vi "CODMn报警信息.vi"(11 "报警簇":T1) -> (3 "CODMN报警信息":string)   [LabVIEW 2016, in "斯坦道CODMn.lvlib"]
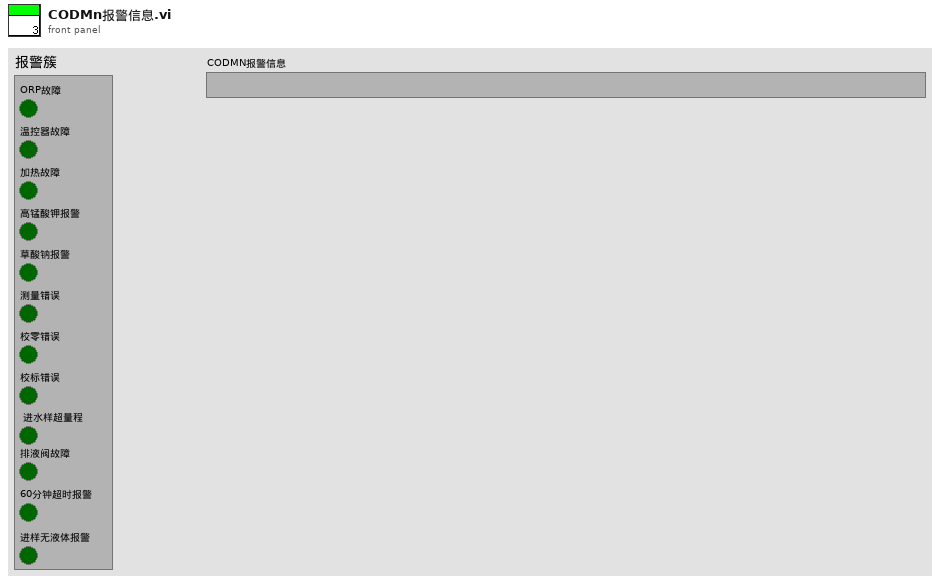
[diagram p1: front panel]
types:
  T1 = cluster{"ORP故障":bool, "温控器故障":bool, "加热故障":bool, "高锰酸钾报警":bool, "草酸钠报警":bool, "测量错误":bool, "校零错误":bool, "校标错误":bool, " 进水样超量程":bool, "排液阀故障":bool, "60分钟超时报警":bool, "进样无液体报警":bool}
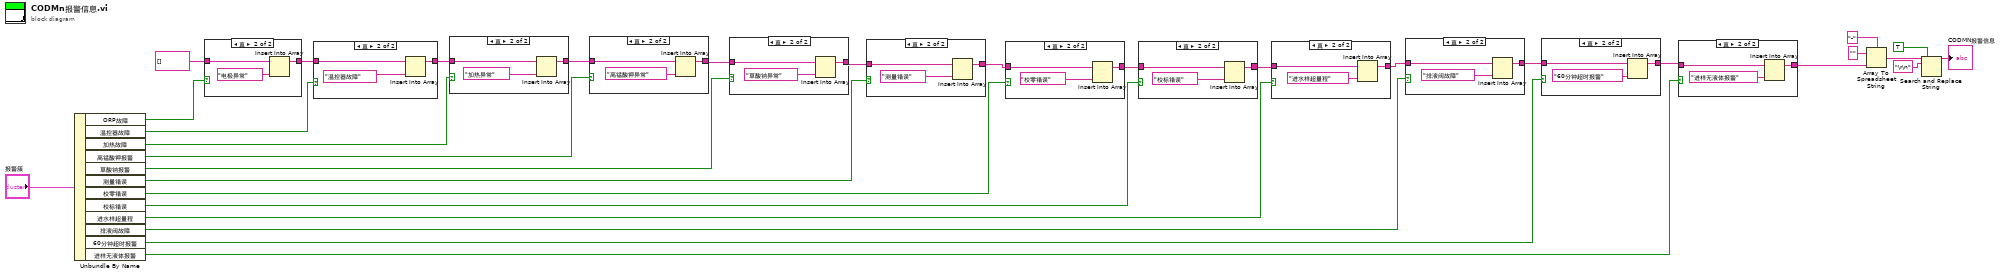
[diagram p0: block diagram]
diagram:
  n1 = Unbundle By Name("报警簇") -> ("ORP故障"=w32:bool, "温控器故障"=w31:bool, "加热故障"=w28:bool, "高锰酸钾报警"=w12:bool, "草酸钠报警"=w11:bool, "测量错误"=w10:bool, "校零错误"=w9:bool, "校标错误"=w8:bool, "进水样超量程"=w7:bool, "排液阀故障"=w6:bool, "60分钟超时报警"=w4:bool, "进样无液体报警"=w2:bool)
  n2 = case shown="真" w32 {
    tunnel: string[] [] -> [w33 w35]
    tunnel: [w33 w34] -> w29
    frame False {
    }
    frame True {
      n3 = Insert Into Array(array=w35, new element="电极异常" ("组合框")) -> (w34:string[])  [unwired: 1 in]
    }
  }
  n4 = case shown="真" w31 {
    tunnel: w29 -> [w37 w40]
    tunnel: [w37 w39] -> w25
    frame False {
    }
    frame True {
      n5 = Insert Into Array(array=w40, new element="温控器故障" ("组合框")) -> (w39:string[])  [unwired: 1 in]
    }
  }
  n6 = case shown="真" w28 {
    tunnel: w25 -> [w41 w43]
    tunnel: [w41 w44] -> w13
    frame False {
    }
    frame True {
      n7 = Insert Into Array(array=w43, new element="加热异常" ("组合框")) -> (w44:string[])  [unwired: 1 in]
    }
  }
  n8 = case shown="真" w12 {
    tunnel: w13 -> [w45 w47]
    tunnel: [w45 w48] -> w14
    frame False {
    }
    frame True {
      n9 = Insert Into Array(array=w47, new element="高锰酸钾异常" ("组合框")) -> (w48:string[])  [unwired: 1 in]
    }
  }
  n10 = case shown="真" w11 {
    tunnel: w14 -> [w49 w51]
    tunnel: [w49 w52] -> w15
    frame False {
    }
    frame True {
      n11 = Insert Into Array(array=w51, new element="草酸钠异常" ("组合框")) -> (w52:string[])  [unwired: 1 in]
    }
  }
  n12 = case shown="真" w10 {
    tunnel: w15 -> [w53 w55]
    tunnel: [w53 w56] -> w16
    frame False {
    }
    frame True {
      n13 = Insert Into Array(array=w55, new element="测量错误" ("组合框")) -> (w56:string[])  [unwired: 1 in]
    }
  }
  n14 = case shown="真" w9 {
    tunnel: w16 -> [w57 w59]
    tunnel: [w57 w60] -> w19
    frame False {
    }
    frame True {
      n15 = Insert Into Array(array=w59, new element="校零错误" ("组合框")) -> (w60:string[])  [unwired: 1 in]
    }
  }
  n16 = case shown="真" w8 {
    tunnel: w19 -> [w61 w63]
    tunnel: [w61 w64] -> w18
    frame False {
    }
    frame True {
      n17 = Insert Into Array(array=w63, new element="校标错误" ("组合框")) -> (w64:string[])  [unwired: 1 in]
    }
  }
  n18 = case shown="真" w7 {
    tunnel: w18 -> [w65 w67]
    tunnel: [w65 w68] -> w17
    frame False {
    }
    frame True {
      n19 = Insert Into Array(array=w67, new element="进水样超量程" ("组合框")) -> (w68:string[])  [unwired: 1 in]
    }
  }
  n20 = case shown="真" w6 {
    tunnel: w17 -> [w69 w71]
    tunnel: [w69 w72] -> w5
    frame False {
    }
    frame True {
      n21 = Insert Into Array(array=w71, new element="排液阀故障" ("组合框")) -> (w72:string[])  [unwired: 1 in]
    }
  }
  n22 = case shown="真" w4 {
    tunnel: w5 -> [w73 w74]
    tunnel: [w73 w76] -> w3
    frame False {
    }
    frame True {
      n23 = Insert Into Array(array=w74, new element="60分钟超时报警" ("组合框")) -> (w76:string[])  [unwired: 1 in]
    }
  }
  n24 = case shown="真" w2 {
    tunnel: w3 -> [w77 w78]
    tunnel: [w77 w80] -> w1
    frame False {
    }
    frame True {
      n25 = Insert Into Array(array=w78, new element="进样无液体报警" ("组合框")) -> (w80:string[])  [unwired: 1 in]
    }
  }
  n26 = Array To Spreadsheet String(delimiter (Tab)="-" ("分隔符(Tab)"), array=w1, 3:"" ("格式字符串")) -> (spreadsheet string=w22:string)
  n27 = Search and Replace String(replace all?=TRUE ("替换全部？(F)"), input string=w22, search string="\r\n" ("搜索字符串")) -> (result string=→"CODMN报警信息":string)  [unwired: 5 in, 3 out]
